vi "UsrProfiles-Prevent profile name dupl.vi"(9 "Profile name ref":refnum<vi>, 10 "New user":bool, 11 "OK button ref":refnum<vi>) -> ()   [LabVIEW 2017]
panel:
  out "Profile name":string
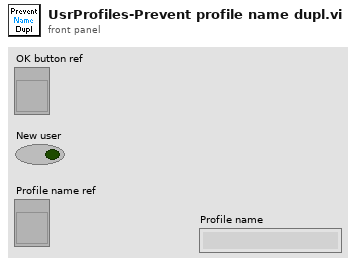
[diagram p1: front panel]
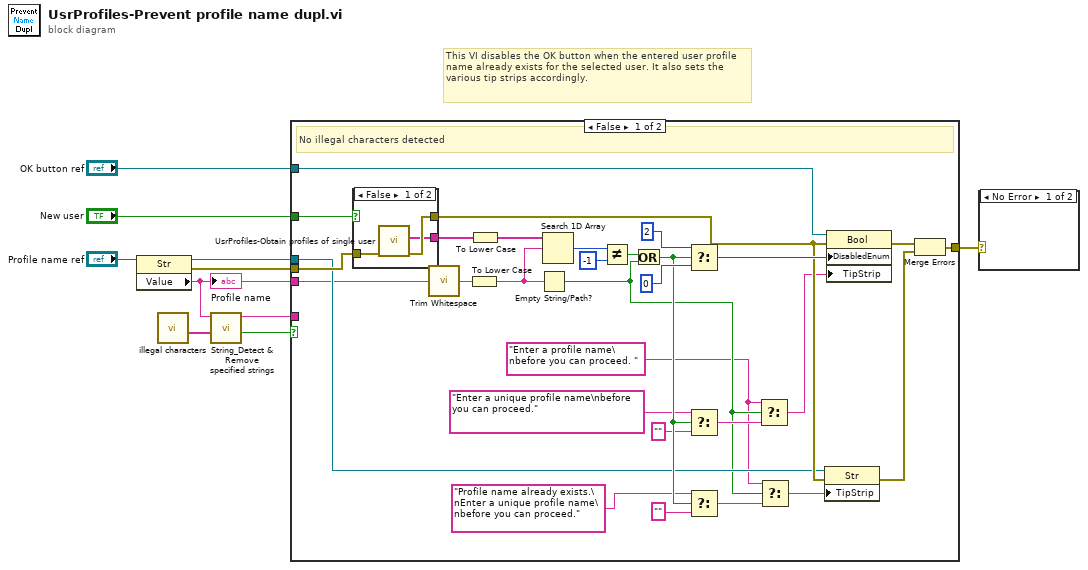
[diagram p0: block diagram]
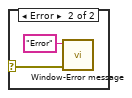
[diagram p2: hidden frame]
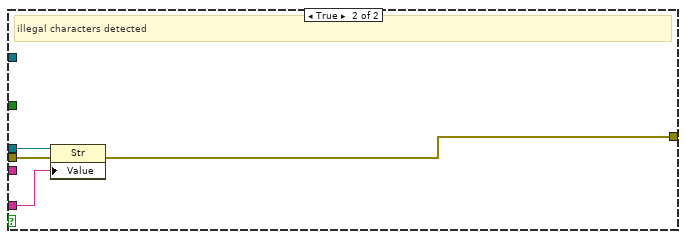
[diagram p4: hidden frame]
diagram:
  # "This VI disables the OK button when the entered user profile name already exists for the selected user. It also sets the various tip strips accordingly."
  n1 = property on="Property Node" class="Str"(reference="Profile name ref") -> (reference out=w7:refnum<vi>, error out=w8:errorcluster, "Value"=w4:string)  [unwired: 1 in]
  "Profile name" <- w4
  n2 = call "illegal characters.vi"() -> ("Array of illegal characters"=w5:string[])  [unwired: 11 in]
  n3 = call <userlib>:"String_Detect & Remove specified strings.vi"("Array of illegal characters or whole words"=w5, "Input string"=w4) -> ("Illegal string detected"=w3:bool, "String with illegal elements removed"=w2:string)  [unwired: 8 in]
  n4 = case shown="False" w3 {
    tunnel: "OK button ref" -> [w34 _]
    tunnel: w8 -> [w33 w46]
    tunnel: w7 -> [w26 w48]
    tunnel: [w23 w45] -> w1
    tunnel: "New user" -> [w12 _]
    tunnel: w4 -> [w11 _]
    tunnel: w2 -> [_ w47]
    frame False {
      w17 = "Enter a profile name\nbefore you can proceed. " ("f")
      # "No illegal characters detected"
      n5 = case shown="False" w12 {
        tunnel: w33 -> [w43 w44]
        tunnel: [w42 w44] -> w27
        tunnel: [w41 _] -> w14
        frame False {
          n6 = call "UsrProfiles-Obtain profiles of single user.vi"("error in"=w43) -> ("error out"=w42:errorcluster, "User profile names"=w41:string[])  [unwired: 9 in]
        }
        frame True {
        }
      }
      n7 = call <vilib>:"Trim Whitespace.vi"("string"=w11) -> ("trimmed string"=w16:string)  [unwired: 1 in]
      n8 = To Lower Case(string=w16) -> (all lower case string=w15:string)
      n9 = To Lower Case(string=w14) -> (all lower case string=w13:string[])
      n10 = Empty String/Path?(string/path=w15) -> (empty?=w18:bool)
      n11 = Search 1D Array(1D array=w13, element=w15) -> (index of element=w35:i32)  [unwired: 1 in]
      n12 = Not Equal?(x=w35, y=-1) -> (x != y?=w37:bool)
      n13 = Or(x=w37, y=w18) -> (x .or. y?=w32:bool)
      n14 = Select(t=2, s=w32, f=0) -> (s? t:f=w38:i32)
      n15 = Select(t="Enter a unique profile name\nbefore you can proceed." ("Profile name"), s=w32, f="") -> (s? t:f=w20:string)
      n16 = Select(t="Profile name already exists.\nEnter a unique profile name\nbefore you can proceed." ("Profile name"), s=w32, f="") -> (s? t:f=w22:string)
      n17 = Select(t=w17, s=w18, f=w20) -> (s? t:f=w19:string)
      n18 = Select(t=w17, s=w18, f=w22) -> (s? t:f=w21:string)
      n19 = property on="Property Node" class="Str"(reference=w26, error in=w27, "TipStrip"=w21) -> (error out=w24:errorcluster)  [unwired: 1 out]
      n20 = property on="Property Node" class="Bool"(reference=w34, error in=w27, "DisabledEnum"=w38, "TipStrip"=w19) -> (error out=w25:errorcluster)  [unwired: 1 out]
      n21 = Merge Errors(w25, w24) -> (w23:errorcluster)
    }
    frame True {
      # "illegal characters detected"
      n22 = property class="Str"(reference=w48, error in=w46, "Value"=w47) -> (error out=w45:errorcluster)  [unwired: 1 out]
    }
  }
  n23 = case shown="No Error" w1 {
    selector: w1 -> [_ w50]
    frame No Error {
    }
    frame Error {
      n24 = call "Window-Error message.vi"("error in (no error)"=w50, "Message"="Error") -> ()  [unwired: 9 in, 1 out]
    }
  }
